vi "CRYASIOStartChannels.vi"(11 "error in (no error)":errorcluster) -> (0 "bResult":bool, 3 "error out":errorcluster)   [LabVIEW 2013]
uses:
  CRY_ASIO.dll
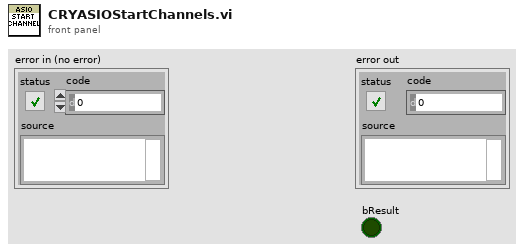
[diagram p1: front panel]
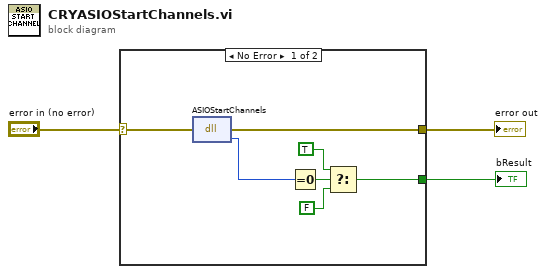
[diagram p0: block diagram]
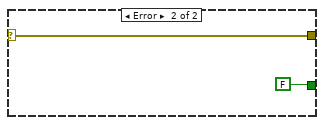
[diagram p2: hidden frame]
diagram:
  n1 = case shown="No Error" "error in (no error)" {
    selector: "error in (no error)" -> [w6 w12]
    tunnel: [w5 w12] -> w2
    tunnel: [w7 FALSE] -> w1
    frame No Error {
      n2 = dll-call lib="D:/LabView_Project/CRY6181/CRY_ASIO.dll" fn="ASIOStartChannels"(error in=w6) -> (error out=w5:errorcluster, "return type"=w4:u32)  [unwired: 2 in, 1 out]
      n3 = Equal To 0?(x=w4) -> (x = 0?=w10:bool)
      n4 = Select(t=TRUE, s=w10, f=FALSE) -> (s? t:f=w7:bool)
    }
    frame Error {
    }
  }
  "error out" <- w2
  "bResult" <- w1
